vi "eventlog format events list.vi"(8 "error in (no error)":errorcluster, 10 "event log (\"\": load current)":string, 11 "Show Archived Logs? (f)":bool) -> (0 "error out":errorcluster, 1 "Template Keys":T1)   [LabVIEW 2011]
uses:
  ITK EXT/utils/keyedarr.llb/Keyed Array.ctl
  ITK EXT/utils/strutil.llb/Case Matching.ctl
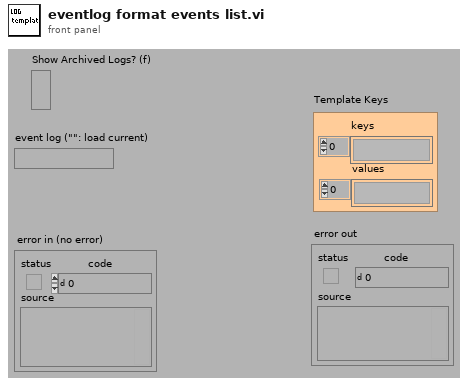
[diagram p1: front panel]
types:
  T1 = typedef "Keyed Array.ctl" = cluster{"keys":string[], "values":string[]}
  T2 = typedef "Case Matching.ctl" = enum16{"a != A", "a == A", "system"}
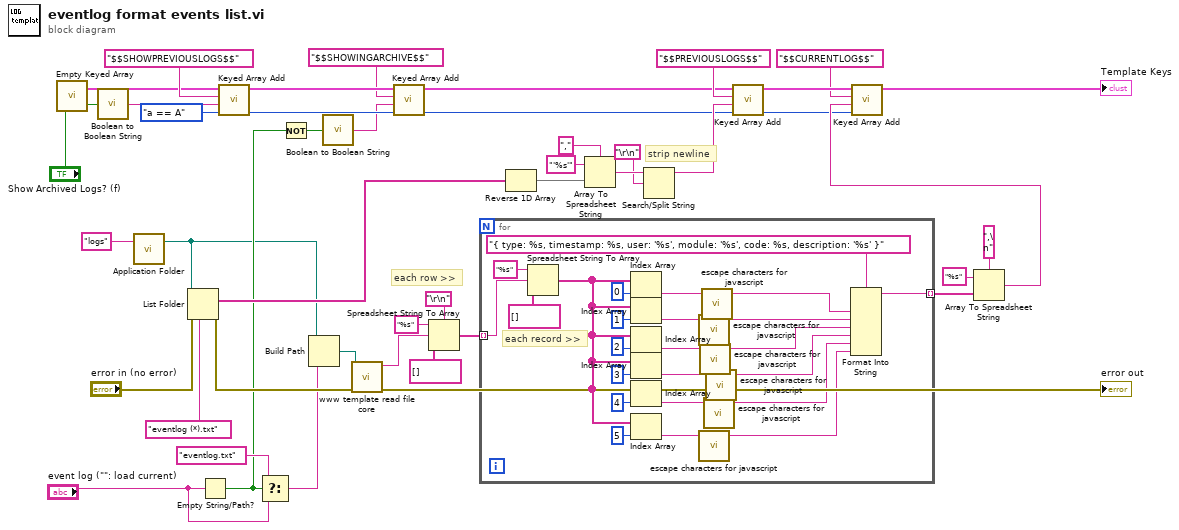
[diagram p0: block diagram]
diagram:
  w8 = Case_Matching."a == A" ("case matching (sensitive)")
  # "each row >>"
  # "strip newline"
  n1 = call "Empty Keyed Array.vi"() -> ("empty keyed array"=w39:T1)  [unwired: 3 out]
  n2 = call "Boolean to Boolean String.vi"("Boolean"="Show Archived Logs? (f)") -> ("Boolean string"=w38:string)  [unwired: 1 in]
  n3 = call "Application Folder.vi"("Relative Path (\"\" - Folder)"="logs" ("format string")) -> ("Application Folder"=w2:path)  [unwired: 2 in]
  n4 = List Folder(path=w2, pattern="eventlog (*).txt" ("format string"), error in="error in (no error)") -> (filenames=w26:string[], error out=w25:errorcluster)  [unwired: 3 out]
  n5 = Empty String/Path?(string/path="event log (\"\": load current)") -> (empty?=w7:bool)
  n6 = call "Keyed Array Add.vi"("case matching (sensitive)"=w8, "value"=w38, "key"="$$SHOWPREVIOUSLOGS$$", "array in"=w39) -> ("array out"=w10:T1)  [unwired: 3 out]
  n7 = Select(t="eventlog.txt" ("format string"), s=w7, f="event log (\"\": load current)") -> (s? t:f=w12:string)
  n8 = Not(x=w7) -> (.not. x?=w6:bool)
  n9 = Build Path(base path=w2, name or relative path=w12) -> (appended path=w23:path)
  n10 = call "Boolean to Boolean String.vi"("Boolean"=w6) -> ("Boolean string"=w4:string)  [unwired: 1 in]
  n11 = call "www template read file core.vi"("error in (no error)"=w25, "Path"=w23) -> ("error out"=→"error out":errorcluster, "File Content"=w22:string)  [unwired: 8 out]
  n12 = call "Keyed Array Add.vi"("case matching (sensitive)"=w8, "value"=w4, "key"="$$SHOWINGARCHIVE$$", "array in"=w10) -> ("array out"=w9:T1)  [unwired: 3 out]
  n13 = Spreadsheet String To Array(delimiter (Tab)="\r\n", format string="%s", spreadsheet string=w22, array type (2D Dbl)=string[] []) -> (array=w18:string[])
  n14 = for {
    tunnel: w18 -> [w63] mode=indexing
    tunnel: [w61] -> w17 mode=indexing
    # "each record >>"
    n15 = Spreadsheet String To Array(format string="%s", spreadsheet string=w63, array type (2D Dbl)=string[] []) -> (array=w49:string[])  [unwired: 1 out]
    n16 = Index Array(array=w49, index=0) -> (element=w60:string)
    n17 = Index Array(array=w49, index=1) -> (element=w59:string)
    n18 = Index Array(array=w49, index=2) -> (element=w54:string)
    n19 = Index Array(array=w49, index=3) -> (element=w53:string)
    n20 = Index Array(array=w49, index=4) -> (element=w51:string)
    n21 = Index Array(array=w49, index=5) -> (element=w43:string)
    n22 = call "escape characters for javascript.vi"("String (\"\")"=w59) -> ("escaped String"=w47:string)  [unwired: 4 out]
    n23 = call "escape characters for javascript.vi"("String (\"\")"=w43) -> ("escaped String"=w42:string)  [unwired: 4 out]
    n24 = call "escape characters for javascript.vi"("String (\"\")"=w54) -> ("escaped String"=w46:string)  [unwired: 4 out]
    n25 = call "escape characters for javascript.vi"("String (\"\")"=w60) -> ("escaped String"=w48:string)  [unwired: 4 out]
    n26 = call "escape characters for javascript.vi"("String (\"\")"=w51) -> ("escaped String"=w44:string)  [unwired: 4 out]
    n27 = call "escape characters for javascript.vi"("String (\"\")"=w53) -> ("escaped String"=w45:string)  [unwired: 4 out]
    n28 = Format Into String(format string="{ type: %s, timestamp: %s, user: '%s', module: '%s', code: %s, description: '%s' }", w48, w47, w46, w45, w44, w42) -> (resulting string=w61:string)  [unwired: 2 in, 1 out]
  }
  n29 = Reverse 1D Array(array=w26) -> (reversed array=w3:string[])
  n30 = Array To Spreadsheet String(delimiter (Tab)=",", array=w3, 3:"'%s'" ("format string")) -> (spreadsheet string=w34:string)
  n31 = Search/Split String(string=w34, search string/char (-)="\r\n") -> (substring before match=w32:string)  [unwired: 3 out]
  n32 = call "Keyed Array Add.vi"("case matching (sensitive)"=w8, "value"=w32, "key"="$$PREVIOUSLOGS$$", "array in"=w9) -> ("array out"=w31:T1)  [unwired: 3 out]
  n33 = Array To Spreadsheet String(delimiter (Tab)=",\n", array=w17, 3:"%s" ("format string")) -> (spreadsheet string=w14:string)
  n34 = call "Keyed Array Add.vi"("case matching (sensitive)"=w8, "value"=w14, "key"="$$CURRENTLOG$$", "array in"=w31) -> ("array out"=→"Template Keys":T1)  [unwired: 3 out]
